vi "Edit DID.vi"(8 "error in (no error)":errorcluster, 11 "Node Ptr":u64 format="%.0x") -> (0 "error out":errorcluster)   [LabVIEW 2015, in "Diagnostics Addon System Explorer.lvlib"]
uses:
  Diagnostics Addon System Explorer.lvlib
  Shared/DIDPID ID FG.vi
  Shared/Get Signals from DIDPID.vi
  Shared/Signal Parameters FG.vi
  Shared/GUID Lookup.vi
  <vilib>/NI Veristand/Custom Device API/Set Item Property (Variant).vi
  <vilib>/NI Veristand/Custom Device API/NI VeriStand - Get Item Property.vi
  <vilib>/NI Veristand/Custom Device API/Get Item Property (Variant).vi
  <vilib>/NI Veristand/Custom Device API/NI VeriStand - Get Item Description.vi
  <vilib>/NI Veristand/Custom Device API/NI VeriStand - Get Custom Device Channel Data.vi
  <vilib>/NI Veristand/Custom Device API/Custom Device API.lvlib
  Shared/Diagnostics Addon Shared.lvlib
  <vilib>/NI Veristand/Custom Device Tools/Custom Device Utility Library/Custom Device Utility Library.lvlib
panel:
  in  "Tag":string
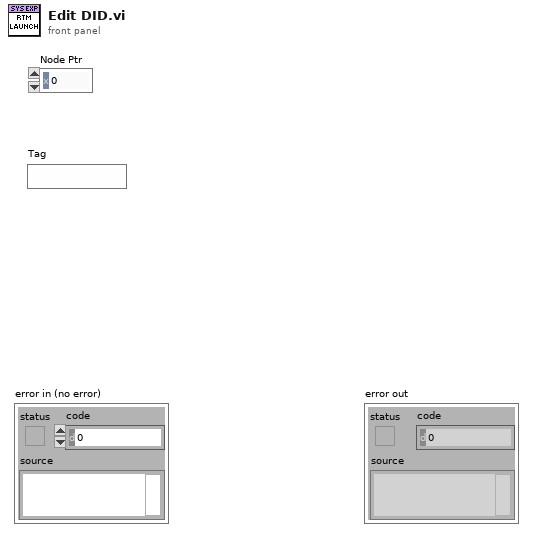
[diagram p1: front panel]
types:
  T1 = typedef "Diagnostics Addon Shared.lvlib/DIDPID Parameters.ctl" = cluster{"Name":string, "Description":string, "ID":u16, "Signals":T2[]}
  T2 = typedef "Diagnostics Addon Shared.lvlib/DIDPID Signal Parameters.ctl" = cluster{"Start Bit":u8, "Length":u8, "Scaling Factor":dbl, "Scaling Offset":dbl, "Minimum":dbl, "Maximum":dbl, "Data Type":u32, "Byte Order":u32, "Default Value":dbl, "Name":string, "Units":string, "Description":string}
  T3 = typedef "Custom Device API.lvlib/Custom Device Item Ref.ctl" = u64
  T4 = typedef "Custom Device API.lvlib/Custom Device Item Info.ctl" = cluster{"Name":string, "Is Channel":bool, "GUID":string, "Is Waveform":bool}
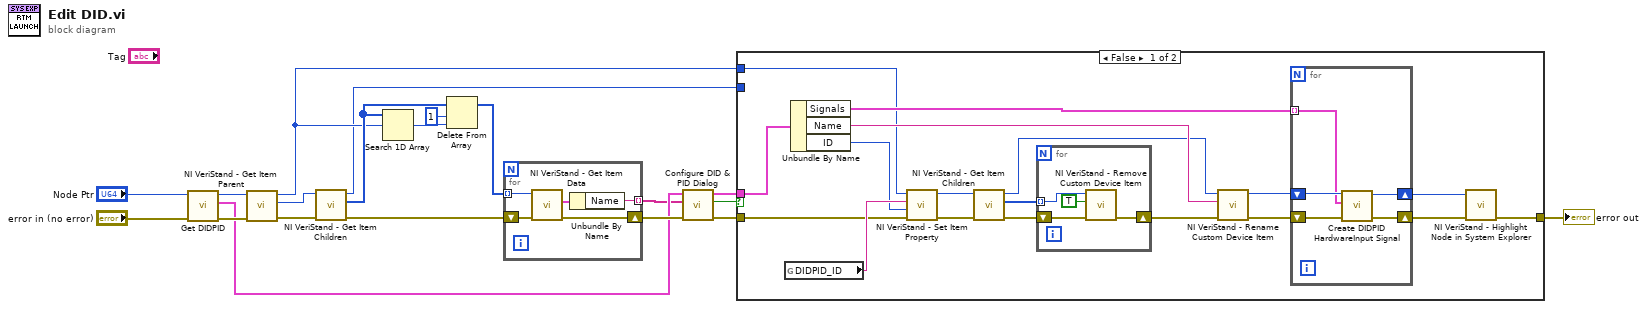
[diagram p0: block diagram]
diagram:
  n1 = call "Get DIDPID.vi"("error in (no error)"="error in (no error)", "Item Ref in"="Node Ptr") -> ("error out"=w8:errorcluster, "PID In"=w5:T1, "Item Ref out"=w6:T3)  [unwired: 7 in]
  n2 = call <vilib>:"NI VeriStand - Get Item Parent.vi"("error in (no error)"=w8, "Item Ref in"=w6) -> ("error out"=w19:errorcluster, "Parent Ref"=w18:T3, "Item Ref out"=w3:T3)  [unwired: 6 in, 1 out]
  n3 = call <vilib>:"NI VeriStand - Get Item Children.vi"("error in (no error)"=w19, "Item Ref in"=w18) -> ("error out"=w20:errorcluster, "Child Refs"=w17:T3[], "Item Ref out"=w2:T3)  [unwired: 6 in, 1 out]
  n4 = Search 1D Array(1D array=w17, element=w3) -> (index of element=w15:i32)  [unwired: 1 in]
  n5 = Delete From Array(array=w17, length=1, index=w15) -> (array with subset deleted=w16:T3[])  [unwired: 1 out]
  n6 = for {
    tunnel: [w23] -> w4 mode=indexing
    shift-right: [w22] -> w10
    shift-left: w20 -> [w24]
    tunnel: w16 -> [w21] mode=indexing
    n7 = call <vilib>:"NI VeriStand - Get Item Data.vi"("error in (no error)"=w24, "Item Ref in"=w21) -> ("error out"=w22:errorcluster, "Item Info"=w25:T4)  [unwired: 8 out]
    n8 = Unbundle By Name(w25) -> ("Name"=w23:string)
  }
  n9 = call "Configure DID & PID Dialog.vi"("error in (no error)"=w10, "Existing PIDs"=w4, "Parameters In"=w5) -> ("error out"=w12:errorcluster, "Cancel PID?"=w11:bool, "Parameters Out"=w13:T1)  [unwired: 6 in]
  n10 = case shown="False" w11 {
    tunnel: w12 -> [w29 w53]
    tunnel: w2 -> [_ _]
    tunnel: w13 -> [w43 _]
    tunnel: [w27 w53] -> w1
    tunnel: w3 -> [w33 _]
    frame False {
      n11 = global read "GUID Lookup.vi" "DIDPID_ID"() -> (w36:string)
      n12 = Unbundle By Name(w43) -> ("Signals"=w39:T2[], "Name"=w42:string, "ID"=w30:u16)
      n13 = call-poly <vilib>:"NI VeriStand - Set Item Property.vi"("error in (no error)"=w29, "Value"=w30, "Property Name"=w36, "Item Ref in"=w33) -> ("error out"=w37:errorcluster, "Item Ref out"=w38:T3)  [unwired: 5 in, 1 out]
      n14 = call <vilib>:"NI VeriStand - Get Item Children.vi"("error in (no error)"=w37, "Item Ref in"=w38) -> ("error out"=w40:errorcluster, "Child Refs"=w41:T3[], "Item Ref out"=w32:T3)  [unwired: 6 in, 1 out]
      n15 = for {
        tunnel: w41 -> [w52] mode=indexing
        shift-right: [w49] -> w35
        shift-left: w40 -> [w51]
        n16 = call <vilib>:"NI VeriStand - Remove Custom Device Item.vi"("error in (no error)"=w51, "Force Delete (F)"=TRUE, "Item Ref in"=w52) -> ("error out"=w49:errorcluster)  [unwired: 7 in, 1 out]
      }
      n17 = call <vilib>:"NI VeriStand - Rename Custom Device Item.vi"("error in (no error)"=w35, "New Name"=w42, "Item Ref in"=w32) -> ("error out"=w34:errorcluster, "Item Ref out"=w31:T3)  [unwired: 1 in, 6 out]
      n18 = for {
        shift-right: [w47] -> w28
        shift-left: w34 -> [w48]
        tunnel: w39 -> [w45] mode=indexing
        shift-right: [w44] -> w26
        shift-left: w31 -> [w46]
        n19 = call "Create DIDPID HardwareInput Signal.vi"("error in (no error)"=w48, "Signal Parameters"=w45, "Section Ptr"=w46) -> ("error out"=w47:errorcluster, "Section Ptr out"=w44:T3)  [unwired: 7 in]
      }
      n20 = call <vilib>:"NI VeriStand - Highlight Node in System Explorer.vi"("error in (no error)"=w28, "Item Ref in"=w26) -> ("error out"=w27:errorcluster)  [unwired: 8 in, 1 out]
    }
    frame True {
    }
  }
  "error out" <- w1
